vi "Read Interlock Values.vi"(8 "error in (no error)":errorcluster, 11 "Simulated Interlocks in":refnum<class "Simulated Interlocks.lvclass">) -> (0 "error out":errorcluster, 2 "Interlock Values":T1)   [LabVIEW 2020, in "Simulated Interlocks.lvclass"]
uses:
  Simulated Interlocks.lvclass
  Door Interlocks/Interlock Values.ctl
  Door Interlocks/Mode of Operation.ctl
  Door Controller/Door Controller/Simulated Values.vi
  Door Interlocks/Door Interlocks.lvclass
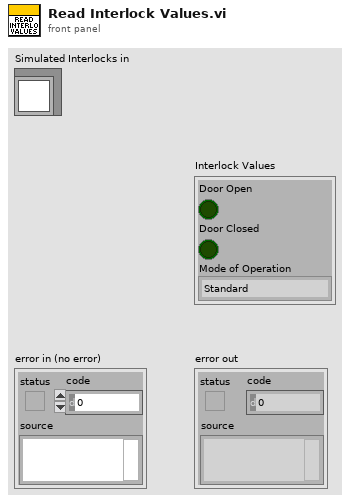
[diagram p1: front panel]
types:
  T1 = typedef "Door Interlocks.lvclass/Interlock Values.ctl" = cluster{"Door Open":bool, "Door Closed":bool, "Mode of Operation":T2}
  T2 = typedef "Door Interlocks.lvclass/Mode of Operation.ctl" = enum16{"Standard", "Interlock Override"}
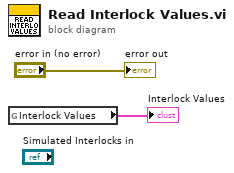
[diagram p0: block diagram]
diagram:
  n1 = global read "Simulated Values.vi" "Interlock Values"() -> (→"Interlock Values":T1)
  "error out" <- "error in (no error)"
